vi "isCompiled.vi"(8 "error in (no error)":errorcluster, 10 "Path":path, 11 "Compiler in":refnum<class "Compiler.lvclass">) -> (0 "error out":errorcluster, 2 "compiled?":bool, 3 "Compiler out":refnum<class "Compiler.lvclass">)   [LabVIEW 2011, in "Compiler.lvlib" / "Compiler.lvclass"]
uses:
  Compiler.lvclass
  Compiler.lvclass/Compiler.ctl
panel:
  out "CompiledPaths":cluster{path, "lastCompiled":timestamp}[](array[cluster])
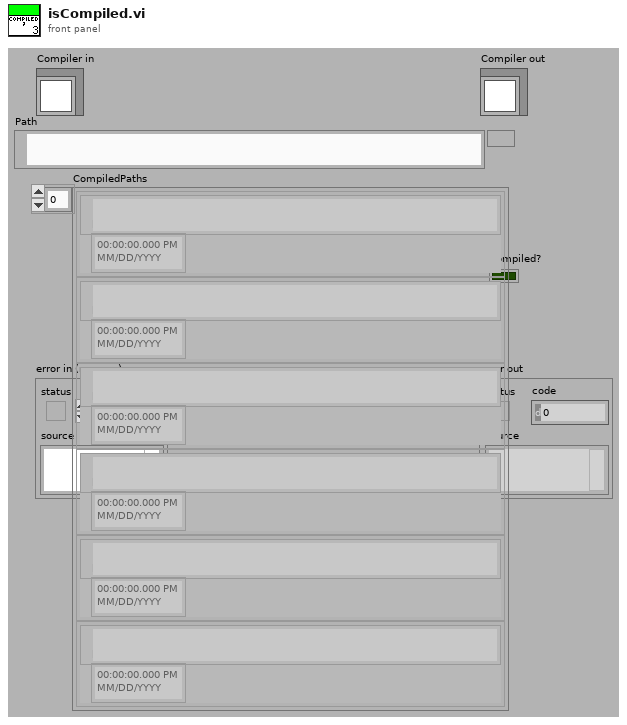
[diagram p1: front panel]
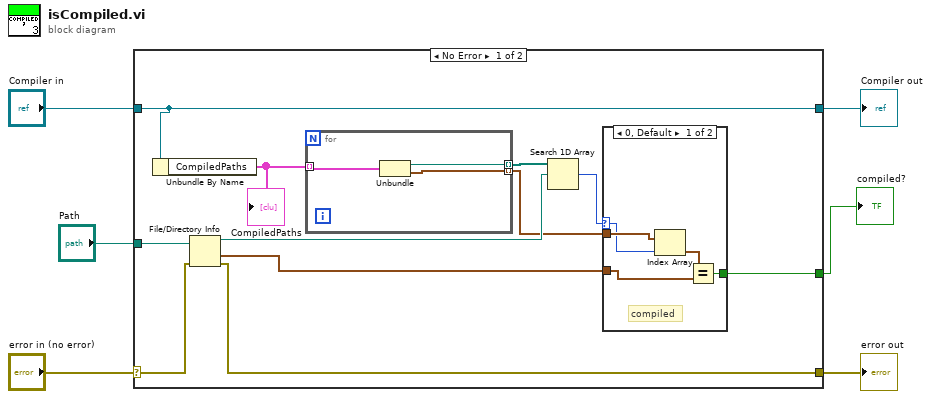
[diagram p0: block diagram]
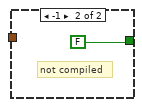
[diagram p2: hidden frame]
diagram:
  n1 = case shown="No Error" "error in (no error)" {
    selector: "error in (no error)" -> [w17 w28]
    tunnel: [w7 w28] -> w5
    tunnel: [w16 w27] -> w3
    tunnel: "Compiler in" -> [w16 w27]
    tunnel: "Path" -> [w14 _]
    tunnel: [w8 _] -> w1
    frame No Error {
      n2 = Unbundle By Name(w16) -> ("CompiledPaths"=w15:cluster{path, "lastCompiled":timestamp}[])
      "CompiledPaths" <- w15
      n3 = File/Directory Info(path=w14, error in=w17) -> (path out=w12:path, last mod=w9:timestamp, error out=w7:errorcluster)  [unwired: 4 out]
      n4 = for {
        tunnel: w15 -> [w26] mode=indexing
        tunnel: [w25] -> w10 mode=indexing
        tunnel: [w24] -> w13 mode=indexing
        n5 = Unbundle(w26) -> (w24:path, "lastCompiled"=w25:timestamp)
      }
      n6 = Search 1D Array(1D array=w13, element=w12) -> (index of element=w11:i32)  [unwired: 1 in]
      n7 = case shown="0, Default" w11 {
        selector: w11 -> [w21 _]
        tunnel: w10 -> [w22 _]
        tunnel: w9 -> [w19 _]
        tunnel: [w18 FALSE] -> w8
        frame 0, Default {
          # "compiled"
          n8 = Index Array(array=w22, index=w21) -> (element=w20:timestamp)
          n9 = Equal?(x=w20, y=w19) -> (x = y?=w18:bool)
        }
        frame -1 {
          # "not compiled"
        }
      }
    }
    frame Error {
    }
  }
  "error out" <- w5
  "Compiler out" <- w3
  "compiled?" <- w1
